vi "encoder_sample_.vi"() -> ()   [LabVIEW 2017]
uses:
  <vilib>/DAQmx/create/channels.llb/DAQmx Create Channel (CI-Position-Angular Encoder).vi
  <resource>/objmgr/daqmx.rc
  <vilib>/DAQmx/read.llb/DAQmx Read (Counter DBL 1Chan 1Samp).vi
panel:
  in  "stop":bool
  out "Waveform Chart":dbl(graph)
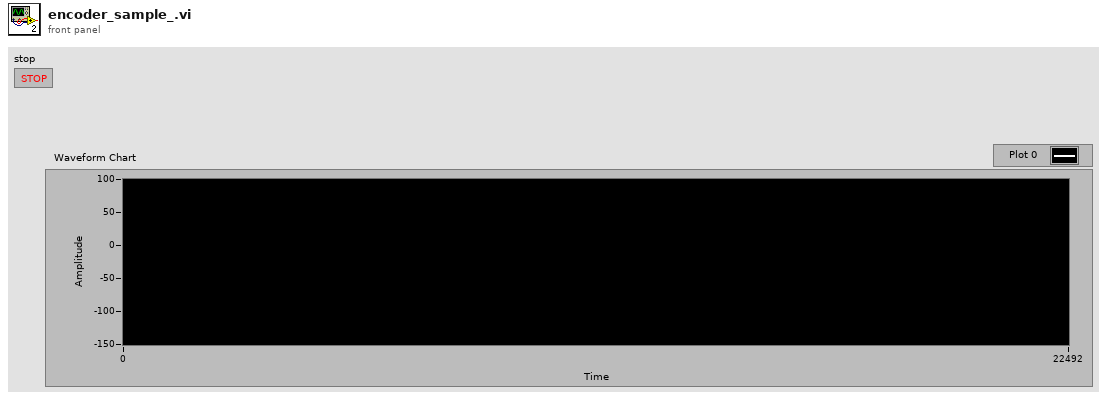
[diagram p1: front panel]
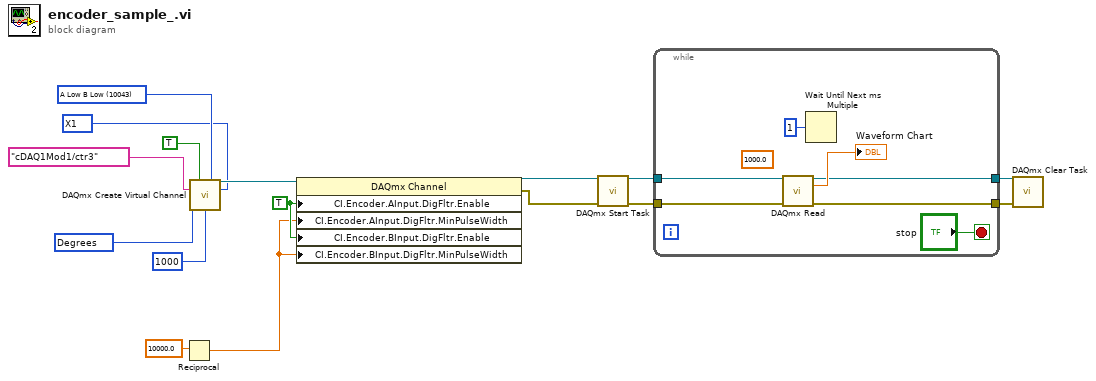
[diagram p0: block diagram]
diagram:
  w9 = TRUE ("CI.Encoder.AInput.DigFltr.Enable")
  w10 = 10090 items=["X1"=10090, "X2"=10091, "X4"=10092, "Two Pulse Counting"=10313] ("decoding type")
  w12 = 10146 items=["Degrees"=10146, "Radians"=10273, "Ticks"=10304, "From Custom Scale"=10065] ("units")
  w14 = 10043 items=["A High B High"=10040, "A High B Low"=10041, "A Low B High"=10042, "A Low B Low"=10043] ("z index phase")
  n1 = Reciprocal(x=10000.0) -> (1/x=w7:dbl)
  n2 = call-poly <vilib>:"DAQmx Create Virtual Channel.vi"("z index enable"=TRUE, "z index phase"=w14, "counter"=tag "cDAQ1Mod1/ctr3", "decoding type"=w10, "units"=w12, "pulses per revolution"=u32 1000) -> ("task out"=w11:refnum<k21>)  [unwired: 8 in, 1 out]
  n3 = property class="DAQmx Channel"(reference=w11, "CI.Encoder.AInput.DigFltr.Enable"=w9, "CI.Encoder.AInput.DigFltr.MinPulseWidth"=w7, "CI.Encoder.BInput.DigFltr.Enable"=w9, "CI.Encoder.BInput.DigFltr.MinPulseWidth"=w7) -> (reference out=w4:refnum<k21>, error out=w3:errorcluster)  [unwired: 1 in]
  n4 = call <vilib>:"DAQmx Start Task.vi"("task/channels in"=w4, "error in"=w3) -> ("task out"=w6:refnum<k21>, "error out"=w5:errorcluster)  [unwired: 12 in]
  n5 = while {
    tunnel: w6 -> [w22]
    tunnel: w5 -> [w21]
    tunnel: [w20] -> w1
    tunnel: [w19] -> w2
    stop <- "stop" stop-if-true
    (unwired) 1000.0 ("timeout")
    n6 = call-poly <vilib>:"DAQmx Read.vi"("task/channels in"=w22, "error in"=w21) -> ("task out"=w19:refnum<k21>, "data"=→"Waveform Chart":dbl, "error out"=w20:errorcluster)  [unwired: 11 in]
    n7 = Wait Until Next ms Multiple(millisecond multiple=u32 1) -> ()  [unwired: 1 out]
  }
  n8 = call <vilib>:"DAQmx Clear Task.vi"("task in"=w2, "error in"=w1) -> ()  [unwired: 13 in, 1 out]
